vi "Start Generation.vi"(8 "error in":errorcluster, 11 "session In":T2) -> (0 "error out":errorcluster, 3 "session out":T1)   [LabVIEW 2023]
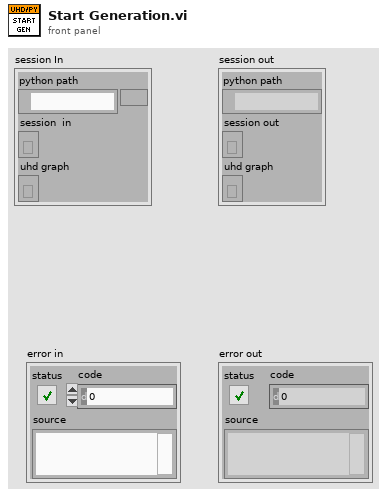
[diagram p1: front panel]
types:
  T1 = cluster{"python path":path, "session out":refnum<k35>, "uhd graph":refnum<k38>}
  T2 = cluster{"python path":path, "session  in":refnum<k35>, "uhd graph":refnum<k38>}
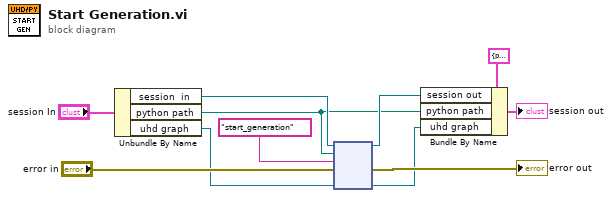
[diagram p0: block diagram]
diagram:
  n1 = Unbundle By Name("session In") -> ("session  in"=w7:refnum<k35>, "python path"=w4:path, "uhd graph"=w3:refnum<k38>)
  n2 = node(w7, w4, "start_generation" ("function name"), "error in", w3) -> (w5:refnum<k35>, →"error out":errorcluster, w2:refnum<k38>)  [unwired: 2 in, 2 out]
  n3 = Bundle By Name(cluster=T1 {"python path"=path "", "session out"=refnum, "uhd graph"=refnum}, "session out"=w5, "python path"=w4, "uhd graph"=w2) -> (→"session out":T1)
